vi "write magnetotropic to file.vi"(0 "g":dbl[](array[numeric])=[3.0, 3.0, 1.0], 1 "jj":dbl[](array[numeric])=[0.0, 0.0], 2 "temperature":dbl(slide)=10.0 scale=0.0..100.0, 3 "Save folder":path=path "/new/data", 4 "spins":enum16{"spin one half", "bipartite"}(ring), 6 "B":dbl[](array[numeric]), 8 "dkdB":dbl[](array[numeric]), 10 "k":dbl[](array[numeric])) -> ()   [LabVIEW 2018]
uses:
  github/resonant_ultrasound_arxiv/maglab ultrasound -- arkady --arxiv/filename-pattern.ctl
  github/resonant_ultrasound_arxiv/maglab ultrasound -- arkady --arxiv/filename-action.ctl
  github/resonant_ultrasound_arxiv/maglab ultrasound -- arkady --arxiv/KM_file -- read-write control.ctl
panel:
  in  "bslope name template":T1={"prefix"="model", "group"="s"}
  in  "bslope file name":string="spin_one_half_g0=3.0_g1=3.0_g2=1.0_J0=0.0_J1=0.0_001_model_051419.dat"
  in  "bsweep name template":T1={"prefix"="model", "group"="b"}
  in  "bsweep file name":string="spin_one_half_g0=3.0_g1=3.0_g2=1.0_J0=0.0_J1=0.0_001_model_051419.dat"
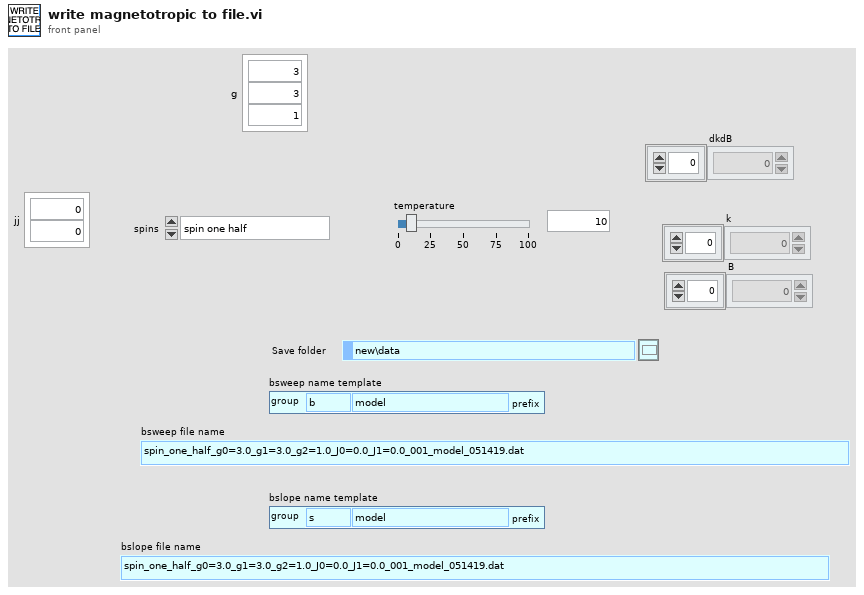
[diagram p1: front panel]
types:
  T1 = typedef "filename-pattern.ctl" = cluster{"prefix":string, "group":string}
  T2 = typedef "KM_file -- read-write control.ctl" = enum16{"read", "write all", "append one line"}
  T3 = typedef "filename-action.ctl" = enum16{"rewrite", "parse", "force pattern", "uniquenum"}
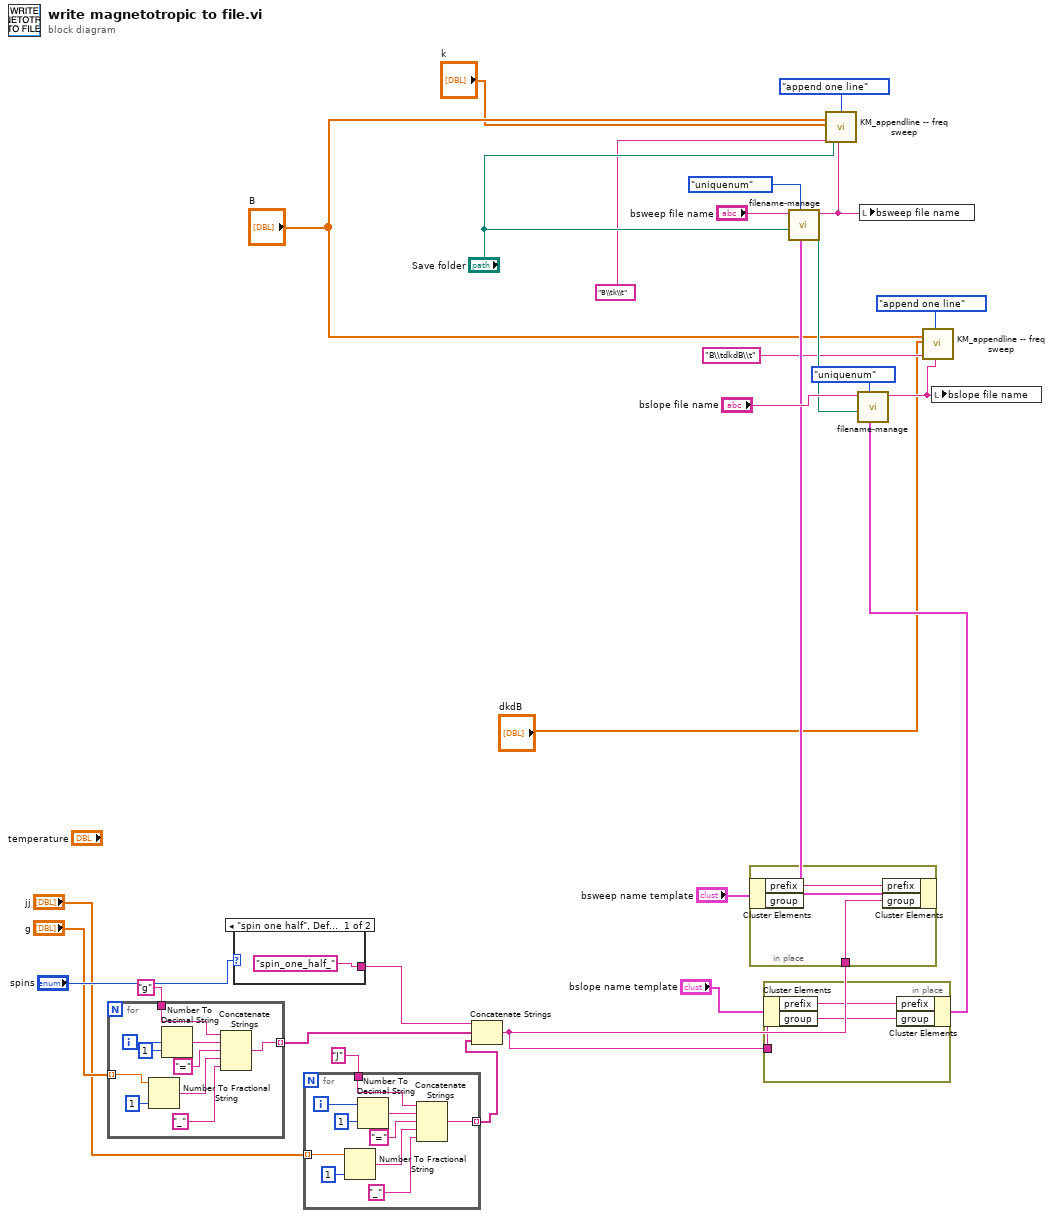
[diagram p0: block diagram]
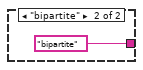
[diagram p2: hidden frame]
diagram:
  n1 = for {
    tunnel: "g" -> [w35] mode=indexing
    tunnel: [w33] -> w14 mode=indexing
    tunnel: "g" -> [w28]
    i -> [w37]
    n2 = Number To Fractional String(number=w35, precision (6)=i16 1) -> (F-format string=w34:string)  [unwired: 2 in]
    n3 = Number To Decimal String(number=w37, width (-)=i16 1) -> (decimal integer string=w36:string)
    n4 = Concatenate Strings(w28, w36, "=", w34, "_") -> (w33:string)
  }
  n5 = case shown="\"spin one half\", Default" "spins" {
    tunnel: ["spin_one_half_" "bipartite"] -> w11
    frame "spin one half", Default {
    }
    frame "bipartite" {
    }
  }
  n6 = for {
    tunnel: "J" -> [w42]
    tunnel: "jj" -> [w41] mode=indexing
    tunnel: [w40] -> w6 mode=indexing
    i -> [w49]
    n7 = Number To Fractional String(number=w41, precision (6)=i16 1) -> (F-format string=w47:string)  [unwired: 2 in]
    n8 = Number To Decimal String(number=w49, width (-)=i16 1) -> (decimal integer string=w48:string)
    n9 = Concatenate Strings(w42, w48, "=", w47, "_") -> (w40:string)
  }
  n10 = Concatenate Strings(w11, w14, w6) -> (w10:string)
  n11 = in-place {
    in-place-border: w10 -> [w50]
    n12 = in-place-cluster #1("bsweep name template") -> ("prefix"=w51:string)  [unwired: 1 out]
    n13 = in-place-cluster #1("prefix"=w51, "group"=w50) -> (w17:T1)
  }
  n14 = in-place {
    in-place-border: w10 -> [w52]
    n15 = in-place-cluster #2("bslope name template") -> ("prefix"=w53:string)  [unwired: 1 out]
    n16 = in-place-cluster #2("prefix"=w53, "group"=w52) -> (w12:T1)
  }
  n17 = call "filename-manage.vi"("filename pattern"=w17, "filename-action"=filename-action."uniquenum", "folder"="Save folder", "file name"="bsweep file name") -> ("filename OUT"=w23:string)  [unwired: 7 in]
  n18 = call "KM_appendline -- freq sweep.vi"("freq"="B", "Vout(V)"="k", "header"="B\\tk\\t", "Save frequency scan"="Save folder", "read/write control"=KM_file_--_read-write_control."append one line", "name or relative path"=w23) -> ()  [unwired: 14 in]
  n19 = call "filename-manage.vi"("filename pattern"=w12, "filename-action"=filename-action."uniquenum", "folder"="Save folder", "file name"="bslope file name") -> ("filename OUT"=w19:string)  [unwired: 7 in]
  n20 = local write "bsweep file name"(w23) -> ()
  n21 = call "KM_appendline -- freq sweep.vi"("freq"="B", "Vout(V)"="dkdB", "header"="B\\tdkdB\\t", "read/write control"=KM_file_--_read-write_control."append one line", "name or relative path"=w19) -> ()  [unwired: 15 in]
  n22 = local write "bslope file name"(w19) -> ()
